vi "HFRR ADV v08.vi"() -> ()   [LabVIEW 2025] (continued)
          frame True {
            (unwired) 0  # existing file
            w3721 = "Choose a datalog file to open"  # prompt
            n2718 = local write "OPEN 3"(FALSE ("OPEN 1")) -> ()
            n2719 = String To Path(string="C:\\LAB-IQ\\Data\\") -> (path=w3706:path)
            n2720 = File Dialog(6:"*.dgf" ("pattern"), 7:w3721, 11:w3706) -> (0:w3704:errorcluster, 3:w3712:path)  [unwired: 4 in, 2 out]
            n2721 = Unbundle(w3704) -> ()  [unwired: 3 out]
            n2722 = Strip Path(path=w3712) -> (name=w3710:string)  [unwired: 1 out]
            n2723 = Path To String(path=w3712) -> (string=w3707:string)
            "string1 3" <- w3707
            n2724 = Match Pattern(string=w3710, regular expression=".dgf") -> (before substring=→"String Control 5":string)  [unwired: 1 in, 3 out]
            n2725 = Match Pattern(string=w3707, regular expression=".dgf" ("substring (\"\")")) -> (before substring=w3717:string)  [unwired: 1 in, 3 out]
            n2726 = Concatenate Strings(w3717, ".duf" ("Substring")) -> (w3714:string)
            n2727 = String To Path(string=w3714) -> (path=w3718:path)
            n2728 = call <vilib>:"Read Characters From File.vi"("file path (dialog if empty)"=w3718, "start of read offset (chars.:0)"=60 ("start of read offset (chars.: 0)")) -> ("character string"=→"String Control 6":string)  [unwired: 4 in, 3 out]
          }
        }
        n2729 = case shown="True" "OPEN 4" {
          frame False {
          }
          frame True {
            (unwired) 0  # existing file
            w3739 = "Choose a datalog file to open"  # prompt
            n2730 = local write "OPEN 4"(FALSE ("OPEN 1")) -> ()
            n2731 = String To Path(string="C:\\LAB-IQ\\Data\\") -> (path=w3724:path)
            n2732 = File Dialog(6:"*.dgf" ("pattern"), 7:w3739, 11:w3724) -> (0:w3722:errorcluster, 3:w3730:path)  [unwired: 4 in, 2 out]
            n2733 = Unbundle(w3722) -> ()  [unwired: 3 out]
            n2734 = Strip Path(path=w3730) -> (name=w3728:string)  [unwired: 1 out]
            n2735 = Path To String(path=w3730) -> (string=w3725:string)
            "string1 4" <- w3725
            n2736 = Match Pattern(string=w3728, regular expression=".dgf") -> (before substring=→"String Control 7":string)  [unwired: 1 in, 3 out]
            n2737 = Match Pattern(string=w3725, regular expression=".dgf" ("substring (\"\")")) -> (before substring=w3735:string)  [unwired: 1 in, 3 out]
            n2738 = Concatenate Strings(w3735, ".duf" ("Substring")) -> (w3732:string)
            n2739 = String To Path(string=w3732) -> (path=w3736:path)
            n2740 = call <vilib>:"Read Characters From File.vi"("file path (dialog if empty)"=w3736, "start of read offset (chars.:0)"=60 ("start of read offset (chars.: 0)")) -> ("character string"=→"String Control 8":string)  [unwired: 4 in, 3 out]
          }
        }
      }
      frame "About" {
        # "Elapsed time\ncof\nstroke\nmean pos\nTemp\nHumidity"
        n2741 = disable-structure shown="Disabled" {
          frame Disabled {
            n2742 = case shown="True" "Export" {
              frame False {
              }
              frame True {
                w3761 = "                                      " ("string")
                w3763 = "\r"
                (unwired) i16 6 ("width (-)")
                w3840 = "\r"
                w3772 = "\r"
                n2743 = local write "Export"(FALSE ("Export")) -> ()
                n2744 = local read "String 29"() -> (w3809:string)
                n2745 = local read "String 34"() -> (w3797:string)
                n2746 = local read "String 35"() -> (w3792:string)
                n2747 = local read "String 37"() -> (w3788:string)
                n2748 = local read "String 36"() -> (w3785:string)
                n2749 = local read "String 38"() -> (w3782:string)
                n2750 = local read "String 39"() -> (w3779:string)
                n2751 = Match Pattern(string=w3809, regular expression=".dwm") -> (before substring=w3805:string)  [unwired: 1 in, 3 out]
                "before substring" <- w3805
                n2752 = local read "S 38"() -> (w3800:string)
                n2753 = local read "S 39"() -> (w3793:string)
                n2754 = local read "Temperature before test 2"() -> (w3829:dbl)
                n2755 = local read "Temperature after test 2"() -> (w3834:dbl)
                n2756 = local read "Humidity before test 2"() -> (w3815:dbl)
                n2757 = local read "Humidity after test 2"() -> (w3830:dbl)
                n2758 = local read "MWSD 2"() -> (w3826:dbl)
                n2759 = local read "WS1.4 2"() -> (w3842:dbl)
                n2760 = local read "HCF 2"() -> (w3838:dbl)
                n2761 = local read "AVP 2"() -> (w3827:dbl)
                n2762 = Concatenate Strings("1," ("string"), w3800) -> (w3799:string)
                n2763 = Concatenate Strings("2," ("string"), w3797) -> (w3796:string)
                n2764 = Concatenate Strings("3," ("string"), w3793) -> (w3795:string)
                n2765 = Concatenate Strings("4," ("string"), w3792) -> (w3791:string)
                n2766 = Concatenate Strings("5," ("string"), w3788) -> (w3789:string)
                n2767 = Concatenate Strings("6," ("string"), w3785) -> (w3786:string)
                n2768 = Concatenate Strings("7," ("string"), w3782) -> (w3783:string)
                n2769 = Concatenate Strings("8," ("string"), w3779) -> (w3780:string)
                n2770 = local read "Sample ID"() -> (w3847:string)
                n2771 = case shown="\"xlx\"" "Select File Type" {
                  tunnel: w3805 -> [w3850 w3852 w3854]
                  tunnel: [w3848 w3853 w3855] -> w3804
                  frame "xlx" {
                    n2772 = Concatenate Strings(w3850, ".xls" ("string")) -> (w3848:string)
                  }
                  frame "csv" {
                    n2773 = Concatenate Strings(w3852, ".csv" ("string")) -> (w3853:string)
                  }
                  frame "txt" {
                    n2774 = Concatenate Strings(w3854, ".txt" ("string")) -> (w3855:string)
                  }
                }
                n2775 = local read "Test Date"() -> (w3846:string)
                n2776 = local read "String 45"() -> (w3760:string)
                n2777 = local read "String 31"() -> (w3845:string)
                n2778 = local read "String 32"() -> (w3844:string)
                n2779 = local read "TITTLE"() -> (w3768:string)
                n2780 = Number To Fractional String(number=w3815, width (-)=i16 6, precision (6)=i16 2) -> (F-format string=w3814:string)  [unwired: 1 in]
                n2781 = Number To Fractional String(number=w3829, width (-)=i16 6, precision (6)=i16 2) -> (F-format string=w3835:string)  [unwired: 1 in]
                n2782 = Number To Fractional String(number=w3830, width (-)=i16 6, precision (6)=i16 2) -> (F-format string=w3828:string)  [unwired: 1 in]
                n2783 = Number To Fractional String(number=w3834, width (-)=i16 6, precision (6)=i16 2) -> (F-format string=w3833:string)  [unwired: 1 in]
                n2784 = Number To Fractional String(number=w3826, width (-)=i16 6, precision (6)=i16 2) -> (F-format string=w3824:string)  [unwired: 1 in]
                n2785 = Number To Fractional String(number=w3827, width (-)=i16 6, precision (6)=i16 2) -> (F-format string=w3825:string)  [unwired: 1 in]
                n2786 = Number To Fractional String(number=w3838, width (-)=i16 6, precision (6)=i16 2) -> (F-format string=w3839:string)  [unwired: 1 in]
                n2787 = Number To Fractional String(number=w3842, precision (6)=i16 2) -> (F-format string=w3843:string)  [unwired: 2 in]
                n2788 = local read "s.NO"() -> (w3762:string)
                n2789 = Concatenate Strings("=" ("string"), w3768) -> (w3767:string)
                n2790 = Concatenate Strings("S.No," ("string"), "                                       Parameters" ("string")) -> (w3773:string)
                n2791 = Concatenate Strings(w3840, w3799, w3814, w3840, w3796, w3835, w3840, w3795, w3828, w3840, w3791, w3833, w3840, w3789, w3824, w3840, w3786, w3825, w3840, w3783, w3839, w3840, w3780, w3843) -> (w3802:string)
                n2792 = Concatenate Strings(w3772, "," ("string"), w3760, w3762, w3761, w3844, w3847, w3761, w3845, w3846, w3772) -> (w3770:string)
                n2793 = local read "Tested by"() -> (w3776:string)
                n2794 = local read "String 33"() -> (w3777:string)
                n2795 = Concatenate Strings("," ("string"), "                                                                             " ("string")) -> (w3765:string)
                n2796 = Concatenate Strings(w3767, w3763, w3770, w3763, w3773, w3802, w3763, w3765, w3777, w3776) -> (→"export":string)
                n2797 = String To Path(string=w3804) -> (path=w3811:path)
                n2798 = local read "export"() -> (w3806:string)
                n2799 = call <vilib>:"Write Characters To File.vi"("append to file? (new file:F)"=FALSE, "character string"=w3806, "file path (dialog if empty)"=w3811) -> ()  [unwired: 2 in, 1 out]
              }
            }
          }
          frame Enabled {
          }
        }
        n2800 = case shown="True" "OK Button 17" {
          frame False {
          }
          frame True {
            (unwired) 0  # existing file
            w4064 = "Choose a datalog file to open"  # prompt
            n2801 = local write "OK Button 17"(FALSE ("OK Button 17")) -> ()
            n2802 = local read "String"() -> (w4059:string)
            n2803 = String To Path(string=w4059) -> (path=w4060:path)
            n2804 = File Dialog(6:"*.duf" ("pattern"), 7:w4064, 11:w4060) -> (0:w4051:errorcluster, 3:w4070:path)  [unwired: 4 in, 2 out]
            n2805 = Unbundle(w4051) -> ()  [unwired: 3 out]
            n2806 = Open/Create/Replace File "Open File"(file path (use dialog)=w4070) -> (refnum out=w4062:refnum<file>)  [unwired: 5 in, 2 out]
            n2807 = Strip Path(path=w4070) -> (name=w4068:string)  [unwired: 1 out]
            n2808 = Path To String(path=w4070) -> (string=w4053:string)
            n2809 = while {
              tunnel: w4062 -> [w4074]
              i -> [w4071]
              stop <- w4072 continue-if-true
              (unwired) TRUE ("line mode (F)")
              n2810 = Read from Text File "Read File"(file (use dialog)=w4074) -> (text=w4073:string)  [unwired: 3 in, 3 out]
              n2811 = local write "Numeric 16"(w4071) -> ()
              n2812 = String Length(string=w4073) -> (length=w4076:i32)
              n2813 = Greater?(x=w4076, y=1) -> (0:w4072:bool)
            }
            n2814 = local write "String 29"(w4053) -> ()
            n2815 = Search and Replace String(input string=w4053, search string=".duf", replace string=".dgf" ("replace string (\"\")")) -> (result string=→"String Indicator 4":string)  [unwired: 5 in, 3 out]
            n2816 = Match Pattern(string=w4068, regular expression=".dwm") -> (before substring=w4052:string)  [unwired: 1 in, 3 out]
            "String Indicator" <- w4052
            n2817 = Match Pattern(string=w4053, regular expression=".dwm" ("substring (\"\")")) -> (before substring=w4054:string)  [unwired: 1 in, 3 out]
            "String Indicator 3" <- w4054
            n2818 = local write "TITTLE 2"(w4052) -> ()
            n2819 = String To Path(string=w4054) -> (path=w4061:path)
            "path" <- w4061
            n2820 = call <vilib>:"Read Characters From File.vi"("file path (dialog if empty)"=w4061, "start of read offset (chars.:0)"=60 ("start of read offset (chars.: 0)")) -> ("character string"=→"String Indicator 2":string)  [unwired: 4 in, 3 out]
          }
        }
        n2821 = call <vilib>:"Query Available Printers.vi"() -> ("system configured printers"=w3753:string[])  [unwired: 9 in, 2 out]
        "System Configured Printers 2" <- w3753
        n2822 = local read "OK Button 16"() -> (w3750:bool)
        n2823 = case shown="True" "OK Button 16" {
          frame False {
          }
          frame True {
            n2824 = stacked-sequence {
              frame #0 {
                n2825 = local read "Numeric 16"() -> (w4078:i32)
                n2826 = local write "Numeric 10"(w4078) -> ()
              }
              frame #1 {
                n2827 = local read "S.NO"() -> (→"s.NO":string)
                n2828 = local read "String 29"() -> (w4082:string)
                n2829 = String To Path(string=w4082) -> (path=w4081:path)
                n2830 = Open/Create/Replace File "Open File"(file path (use dialog)=w4081) -> (refnum out=w4083:refnum<file>)  [unwired: 5 in, 2 out]
                n2831 = for {
                  N: 16 -> [_]
                  tunnel: w4083 -> [w4090]
                  i -> [w4086]
                  (unwired) TRUE ("line mode (F)")
                  n2832 = Read from Text File "Read File"(file (use dialog)=w4090) -> (text=w4084:string)  [unwired: 3 in, 3 out]
                  n2833 = Match Pattern(string=w4084, regular expression="(") -> (after substring=w4089:string)  [unwired: 1 in, 3 out]
                  n2834 = Match Pattern(string=w4089, regular expression=")") -> (before substring=w4085:string)  [unwired: 1 in, 3 out]
                  n2835 = case shown="1" w4086 {
                    tunnel: w4085 -> [w4091 w4092 _ _ w4093 w4094 w4095 w4097 w4099 w4101 w4103 w4105 w4107 w4109 _]
                    tunnel: w4084 -> [_ _ _ _ _ _ _ _ _ _ _ _ _ _ _]
                    frame 0 {
                      "TITTLE" <- w4091
                    }
                    frame 1 {
                      "Sample ID" <- w4092
                    }
                    frame 2 {
                    }
                    frame 3 {
                    }
                    frame 4 {
                      "Test Date" <- w4093
                    }
                    frame 5 {
                      "Tested by" <- w4094
                    }
                    frame 6 {
                      n2836 = Fract/Exp String To Number(string=w4095) -> (number=→"Humidity before test 2":dbl)  [unwired: 3 in, 1 out]
                    }
                    frame 7 {
                      n2837 = Fract/Exp String To Number(string=w4097) -> (number=→"Temperature before test 2":dbl)  [unwired: 3 in, 1 out]
                    }
                    frame 8 {
                      n2838 = Fract/Exp String To Number(string=w4099) -> (number=→"Humidity after test 2":dbl)  [unwired: 3 in, 1 out]
                    }
                    frame 9 {
                      n2839 = Fract/Exp String To Number(string=w4101) -> (number=→"Temperature after test 2":dbl)  [unwired: 3 in, 1 out]
                    }
                    frame 10 {
                      n2840 = Fract/Exp String To Number(string=w4103) -> (number=→"MWSD 2":dbl)  [unwired: 3 in, 1 out]
                    }
                    frame 11 {
                      n2841 = Fract/Exp String To Number(string=w4105) -> (number=→"AVP 2":dbl)  [unwired: 3 in, 1 out]
                    }
                    frame 12 {
                      n2842 = Fract/Exp String To Number(string=w4107) -> (number=→"HCF 2":dbl)  [unwired: 3 in, 1 out]
                    }
                    frame 13 {
                      n2843 = Fract/Exp String To Number(string=w4109) -> (number=→"WS1.4 2":dbl)  [unwired: 3 in, 1 out]
                    }
                    frame 14, Default {
                    }
                  }
                }
              }
              frame #2 {
              }
            }
            n2844 = local write "OK Button 16"(FALSE ("OK Button 13")) -> ()
          }
        }
        n2845 = Index Array(array=w3753, index="Select Printer 3") -> (element=w3755:string)
        "Selected Printer" <- w3755
        n2846 = case shown="True" w3750 {
          frame False {
          }
          frame True {
            n2847 = flat-sequence {
              frame #0 {
              }
              frame #1 {
                n2848 = Wait (ms)(milliseconds to wait=u32 100) -> ()  [unwired: 1 out]
              }
              frame #2 {
                n2849 = local write "OK Button 16"(FALSE ("Print 3")) -> ()
              }
            }
          }
        }
        n2850 = case shown="True" "Print" {
          tunnel: w3755 -> [_ w4047]
          frame False {
          }
          frame True {
            (unwired) i16 6 ("width (-)")
            (unwired) "TESTED BY : "
            (unwired) "TESTED DATE :"
            (unwired) "SAMPLE ID : "
            (unwired) "SAMPLE DESIGN : "
            w4005 = "\r"
            w4022 = "\r"
            # "add image"
            n2851 = local read "Sample ID"() -> (w3995:string)
            n2852 = local read "Tested by"() -> (w3998:string)
            n2853 = local read "String 34"() -> (w3985:string)
            n2854 = local read "String 45"() -> (w3965:string)
            n2855 = local read "String 35"() -> (w3980:string)
            n2856 = local read "String 37"() -> (w3978:string)
            n2857 = local read "String 32"() -> (w4000:string)
            n2858 = local read "String 36"() -> (w3975:string)
            n2859 = local read "String 31"() -> (w3999:string)
            n2860 = local read "Test Date"() -> (w3996:string)
            n2861 = local read "String 33"() -> (w4001:string)
            n2862 = local read "String 38"() -> (w3971:string)
            n2863 = local read "String 39"() -> (w3968:string)
            n2864 = local write "Print"(FALSE ("Print FF")) -> ()
            n2865 = local read "S 39"() -> (w3983:string)
            n2866 = local read "S 38"() -> (w3990:string)
            n2867 = local read "Temperature before test 2"() -> (w4021:dbl)
            n2868 = local read "Temperature after test 2"() -> (w4011:dbl)
            n2869 = local read "Humidity before test 2"() -> (w4036:dbl)
            n2870 = local read "Humidity after test 2"() -> (w4020:dbl)
            n2871 = local read "MWSD 2"() -> (w4025:dbl)
            n2872 = local read "WS1.4 2"() -> (w4003:dbl)
            n2873 = Concatenate Strings("2)" ("string"), w3985) -> (w3986:string)
            n2874 = Concatenate Strings("3)" ("string"), w3983) -> (w3984:string)
            n2875 = Concatenate Strings("1)" ("string"), w3990) -> (w3989:string)
            n2876 = Concatenate Strings("4)" ("string"), w3980) -> (w3981:string)
            n2877 = Concatenate Strings("5)" ("string"), w3978) -> (w3977:string)
            n2878 = Concatenate Strings("6)" ("string"), w3975) -> (w3974:string)
            n2879 = Concatenate Strings("7)" ("string"), w3971) -> (w3972:string)
            n2880 = Concatenate Strings("8)" ("string"), w3968) -> (w3969:string)
            n2881 = local read "HCF 2"() -> (w4007:dbl)
            n2882 = local read "AVP 2"() -> (w4024:dbl)
            n2883 = local read "s.NO"() -> (w3966:string)
            n2884 = call <vilib>:"New Report.vi"("report type"=enum16{"Standard Report", "HTML"}."Standard Report") -> ("report out"=w4045:refnum<class "NI_report.lvclass">, "error out"=w4044:errorcluster)  [unwired: 13 in]
            n2885 = local read "TITTLE"() -> (w3997:string)
            n2886 = Concatenate Strings(w4022, w3965, w3966, w4022, w4000, w3995, w4022, w3999, w3996, w4022, w4001, w3998, w4022) -> (w4015:string)
            "test by" <- w4015
            n2887 = Number To Fractional String(number=w4021, width (-)=i16 6, precision (6)=i16 2) -> (F-format string=w4010:string)  [unwired: 1 in]
            n2888 = Number To Fractional String(number=w4020, width (-)=i16 6, precision (6)=i16 2) -> (F-format string=w4023:string)  [unwired: 1 in]
            n2889 = Number To Fractional String(number=w4036, width (-)=i16 6, precision (6)=i16 2) -> (F-format string=w4041:string)  [unwired: 1 in]
            n2890 = Number To Fractional String(number=w4025, width (-)=i16 6, precision (6)=i16 2) -> (F-format string=w4027:string)  [unwired: 1 in]
            n2891 = Number To Fractional String(number=w4011, width (-)=i16 6, precision (6)=i16 2) -> (F-format string=w4012:string)  [unwired: 1 in]
            n2892 = Number To Fractional String(number=w4024, width (-)=i16 6, precision (6)=i16 2) -> (F-format string=w4026:string)  [unwired: 1 in]
            n2893 = Number To Fractional String(number=w4007, width (-)=i16 6, precision (6)=i16 2) -> (F-format string=w4006:string)  [unwired: 1 in]
            n2894 = Number To Fractional String(number=w4003, precision (6)=i16 2) -> (F-format string=w4002:string)  [unwired: 2 in]
            n2895 = call-dynamic "Set Report Header Text.vi"("report in"=w4045, "center header text"=w3997, "error in (no error)"=w4044) -> ("report out"=w4016:refnum<class "NI_report.lvclass">, "error out"=w4017:errorcluster)  [unwired: 11 in]
            n2896 = Concatenate Strings(w4005, w3989, w4041, w4005, w3986, w4010, w4005, w3984, w4023, w4005, w3981, w4012, w4005, w3977, w4027, w4005, w3974, w4026, w4005, w3972, w4006, w4005, w3969, w4002) -> (w3993:string)
            "export 2" <- w3993
            n2897 = call-poly <vilib>:"Append Report Text.vi"("report in"=w4016, "text"=w4015, "error in (no error)"=w4017) -> ("report out"=w4019:refnum<class "NI_report.lvclass">, "error out"=w4018:errorcluster)  [unwired: 9 in, 2 out]
            n2898 = local read "test by"() -> (w3992:string)
            n2899 = local read "TITTLE"() -> (w3994:string)
            n2900 = call-poly <vilib>:"Append Report Text.vi"("report in"=w4019, "error in (no error)"=w4018) -> ("report out"=w4040:refnum<class "NI_report.lvclass">, "error out"=w4038:errorcluster)  [unwired: 10 in, 2 out]
            n2901 = Concatenate Strings(w3994, w3993, w3992) -> (→"output":string)
            n2902 = call-poly <vilib>:"Append Report Text.vi"("report in"=w4040, "text"=w3993, "error in (no error)"=w4038) -> ("report out"=w4039:refnum<class "NI_report.lvclass">, "error out"=w4037:errorcluster)  [unwired: 9 in, 2 out]
            n2903 = call-dynamic "Print Report.vi"("report in"=w4039, "printer name (default)"=w4047, "error in (no error)"=w4037) -> ("report out"=w4049:refnum<class "NI_report.lvclass">, "error out"=w4050:errorcluster)  [unwired: 11 in]
            n2904 = call-dynamic "Dispose Report.vi"("report in"=w4049, "error in (no error)"=w4050) -> ()  [unwired: 13 in, 1 out]
          }
        }
        n2905 = case shown="True" "Print 2" {
          frame False {
          }
          frame True {
            n2906 = flat-sequence {
              frame #0 {
                n2907 = local read "s.NO"() -> (→"s.NO 2":string)
                n2908 = Wait (ms)(milliseconds to wait=u32 20) -> ()  [unwired: 1 out]
                n2909 = local read "Sample ID  3"() -> (→"Sample ID  6":string)
                n2910 = local read "Sample ID  4"() -> (→"Sample ID  7":string)
                n2911 = local read "Sample ID"() -> (→"Sample ID  2":string)
                n2912 = local read "Tested by"() -> (→"Tested by 2":string)
                n2913 = local read "Test Date"() -> (→"Test Date 2":string)
                n2914 = local read "Humidity after test 3"() -> (→"Humidity after test 4":dbl)
                n2915 = local read "Ref A Test Date :"() -> (→"TITTLE 4":string)
                n2916 = local read "Temperature before test 3"() -> (w3872:dbl)
                n2917 = local read "Temperature before test 3"() -> (→"Temperature after test 5":dbl)
                n2918 = local read "Temperature after test 3"() -> (→"Temperature after test 4":dbl)
                n2919 = local read "Humidity before test 3"() -> (→"Humidity before test 4":dbl)
                n2920 = local write "Temperature before test 3"(w3872) -> ()
                n2921 = local read "image data"() -> (w3863:T12)
                n2922 = String To Path(string="C:\\LAB-IQ\\im\\Temp_resized.jpg") -> (path=w3864:path)
                "path 2" <- w3864
                n2923 = call <vilib>:"Write JPEG File.vi"("image data"=w3863, "path to JPEG file"=w3864) -> ()  [unwired: 8 in, 2 out]
                "Ref A Test Date :" <- "Ref A Test Date :"
                "Ref B Test Date :" <- "Ref B Test Date :"
                "Ref B Scar Value :" <- "Ref B Scar Value :"
                "Ref A Scar Value :" <- "Ref A Scar Value :"
              }
              frame #1 {
                (unwired) HTML_Report_Image_Alignment."MIDDLE" ("alignment (default)")
                w3900 = u16 0 items=["portrait", "landscape"] ("orientation (portrait)")
                (unwired) HTML_Report_Image_Alignment."ABSMIDDLE" ("alignment (default)")
                (unwired) "TESTED BY : "
                (unwired) "TESTED DATE :"
                (unwired) "SAMPLE ID : "
                (unwired) "SAMPLE DESIGN : "
                w3933 = "\r"
                # "add image"
                n2924 = Wait (ms)(milliseconds to wait=u32 20) -> ()  [unwired: 1 out]
                n2925 = local read "Sample ID  2"() -> (w3926:string)
                n2926 = local read "Wear Scar X"() -> (w3898:dbl)
                "Length ( microns ) 2" <- w3898
                n2927 = local read "Wear Scar Y"() -> (w3897:dbl)
                "Wear Scar Y ( microns ) :" <- w3897
                n2928 = local read "Test Date 2"() -> (w3927:string)
                n2929 = local read "Tested by 2"() -> (w3928:string)
                n2930 = local read "String 46"() -> (w3924:string)
                n2931 = local read "String 48"() -> (w3930:string)
                n2932 = local read "String 47"() -> (w3929:string)
                n2933 = local read "String 49"() -> (w3931:string)
                n2934 = local read "String 10"() -> (w3884:string)
                n2935 = local read "s.NO 2"() -> (w3925:string)
                n2936 = Add(x=w3898, y=w3897) -> (x+y=w3896:dbl)
                n2937 = call <vilib>:"New Report.vi"("report type"=enum16{"Standard Report", "HTML"}."HTML") -> ("report out"=w3904:refnum<class "NI_report.lvclass">, "error out"=w3902:errorcluster)  [unwired: 13 in]
                n2938 = Concatenate Strings(w3933, w3924, w3925, w3933, w3930, w3926, w3933, w3929, w3927, w3933, w3931, w3928, w3933) -> (→"test by 2":string)
                n2939 = Concatenate Strings("C:\\LAB-IQ\\Data\\" ("string"), w3884, ".jpg" ("string")) -> ()  [unwired: 1 out]
                n2940 = Divide(x=w3896, y=2.0) -> (x/y=→"Mean Wear ( microns) :":dbl)
                n2941 = call-dynamic "Set Report Orientation.vi"("report in"=w3904, "orientation (portrait)"=w3900, "error in (no error)"=w3902) -> ("report out"=w3903:refnum<class "NI_report.lvclass">, "error out"=w3901:errorcluster)  [unwired: 11 in]
                n2942 = for {
                  N: 5 -> [_]
                  tunnel: w3903 -> [w3954]
                  tunnel: [w3953] -> w3882
                  tunnel: w3901 -> [w3952]
                  tunnel: [w3951] -> w3881
                  n2943 = call-dynamic "Set Report Tab Width.vi"("report in"=w3954, "error in (no error)"=w3952) -> ("report out"=w3953:refnum<class "NI_report.lvclass">, "error out"=w3951:errorcluster)  [unwired: 12 in]
                }
                n2944 = local read "TITTLE"() -> (w3899:string)
                n2945 = call-dynamic "Set Report Header Text.vi"("report in"=w3882, "center header text"=w3899, "error in (no error)"=w3881) -> ("report out"=w3920:refnum<class "NI_report.lvclass">, "error out"=w3919:errorcluster)  [unwired: 11 in]
                n2946 = for {
                  N: 1 -> [_]
                  tunnel: [w3958] -> w3906
                  tunnel: [w3957] -> w3905
                  tunnel: w3920 -> [w3956]
                  tunnel: w3919 -> [w3955]
                  n2947 = call-dynamic "New Report Line.vi"("report in"=w3956, "error in (no error)"=w3955) -> ("report out"=w3958:refnum<class "NI_report.lvclass">, "error out"=w3957:errorcluster)  [unwired: 12 in]
                }
                n2948 = for {
                  N: 2 -> [_]
                  tunnel: [w3950] -> w3912
                  tunnel: [w3949] -> w3911
                  tunnel: w3906 -> [w3948]
                  tunnel: w3905 -> [w3947]
                  n2949 = call-dynamic "New Report Line.vi"("report in"=w3948, "error in (no error)"=w3947) -> ("report out"=w3950:refnum<class "NI_report.lvclass">, "error out"=w3949:errorcluster)  [unwired: 12 in]
                }
                n2950 = for {
                  N: 25 -> [_]
                  tunnel: w3912 -> [w3946]
                  tunnel: w3911 -> [w3944]
                  tunnel: [w3945] -> w3915
                  tunnel: [w3943] -> w3914
                  n2951 = call-dynamic "Set Report Tab Width.vi"("report in"=w3946, "error in (no error)"=w3944) -> ("report out"=w3945:refnum<class "NI_report.lvclass">, "error out"=w3943:errorcluster)  [unwired: 12 in]
                }
                n2952 = control-ref of="Tab Control 9"() -> (w3910:refnum<vi>)
                n2953 = call-dynamic "Append Control Image to Report.vi"("report in"=w3915, "alignment (default)"=HTML_Report_Image_Alignment."ABSMIDDLE", "ctrl reference"=w3910, "error in (no error)"=w3914) -> ("report out"=w3909:refnum<class "NI_report.lvclass">, "error out"=w3908:errorcluster)  [unwired: 8 in, 2 out]
                n2954 = for {
                  N: 3 -> [_]
                  tunnel: [w3942] -> w3893
                  tunnel: [w3941] -> w3892
                  tunnel: w3909 -> [w3940]
                  tunnel: w3908 -> [w3939]
                  n2955 = call-dynamic "New Report Line.vi"("report in"=w3940, "error in (no error)"=w3939) -> ("report out"=w3942:refnum<class "NI_report.lvclass">, "error out"=w3941:errorcluster)  [unwired: 12 in]
                }
                n2956 = for {
                  N: 100 -> [_]
                  tunnel: w3893 -> [w3938]
                  tunnel: w3892 -> [w3936]
                  tunnel: [w3937] -> w3889
                  tunnel: [w3935] -> w3887
                  n2957 = call-dynamic "Set Report Tab Width.vi"("report in"=w3938, "error in (no error)"=w3936) -> ("report out"=w3937:refnum<class "NI_report.lvclass">, "error out"=w3935:errorcluster)  [unwired: 12 in]
                }
                n2958 = String To Path(string="C:\\LAB-IQ\\im\\Temp_resized.jpg") -> (path=w3879:path)
                n2959 = call-poly <vilib>:"Append Image to Report.vi"("report in"=w3889, "path or URL of image"=w3879, "error in (no error)"=w3887) -> ("report out"=w3888:refnum<class "NI_report.lvclass">, "error out"=w3886:errorcluster)  [unwired: 9 in, 2 out]
                n2960 = call-poly <vilib>:"Open HTML Report in Browser.vi"("report in"=w3888, "error in (no error)"=w3886) -> ("report out"=w3923:refnum<class "NI_report.lvclass">, "error out"=w3922:errorcluster)  [unwired: 11 in, 1 out]
                n2961 = call-dynamic "Dispose Report.vi"("report in"=w3923, "error in (no error)"=w3922) -> ()  [unwired: 13 in, 1 out]
              }
              frame #2 {
              }
              frame #3 {
                n2962 = disable-structure shown="Disabled" {
                  frame Disabled {
                    n2963 = local read "String 10"() -> (w3963:string)
                    n2964 = Concatenate Strings("C:\\LAB-IQ-NXT\\Data\\" ("string"), w3963, ".jpg" ("string")) -> (w3961:string)
                    n2965 = String To Path(string=w3961) -> (path=w3960:path)
                    n2966 = Delete(path (use dialog)=w3960) -> ()  [unwired: 4 in, 3 out]
                  }
                  frame Enabled {
                  }
                }
                n2967 = local write "Print 2"(FALSE ("Print")) -> ()
              }
            }
          }
        }
      }
    }
    n2968 = property on="SetTemp" class="DigNum (strict)"("Disabled"=w1894) -> ()  [unwired: 2 in, 2 out]
    n2969 = Multiply(x=w1883, y=w1885) -> (x*y=w1884:dbl)
    n2970 = local read "MWSD"() -> (w1882:dbl)
    n2971 = Add(x=w1884, y=w1882) -> (x+y=→"WS1.4":dbl)
    n2972 = Wait (ms)(milliseconds to wait=u32 50) -> ()  [unwired: 1 out]
    n2973 = Wait (ms)(milliseconds to wait=u32 50) -> ()  [unwired: 1 out]
    n2974 = local read "Quit"() -> (w1881:bool)
  }
  n2975 = VISA Close(VISA resource name=w46, error in (no error)=w45) -> (error out=w43:errorcluster)
  n2976 = VISA Close(VISA resource name=w27, error in (no error)=w26) -> ()  [unwired: 1 out]
  n2977 = call <vilib>:"Clear Errors.vi"("error in (no error)"=w43) -> ()  [unwired: 5 in, 2 out]
  n2978 = Or(x=w33, y=w32) -> (x .or. y?=w34:bool)
  n2979 = while {
    tunnel: [w4111] -> w39
    shift-right: [w4149] -> _
    shift-left: "" -> [w4137]
    tunnel: [w4125] -> _
    i -> [w4125]
    stop <- w4111 stop-if-true
    w4151 = ";" ("string")
    n2980 = local read "start en"() -> (w4170:bool)
    n2981 = And(x="st enable", y=w4170) -> (x .and. y?=w4171:bool)
    n2982 = local read "ACQUIRE 3"() -> (w4114:bool)
    n2983 = local read "Elapsed time"() -> (w4133:dbl)
    n2984 = case shown="True" w4171 {
      tunnel: "st enable" -> [w4235 w4236]
      tunnel: [w4235 w4236] -> w4115
      frame False {
      }
      frame True {
        n2985 = local write "start en"(FALSE ("start en")) -> ()
      }
    }
    n2986 = Wait (ms)(milliseconds to wait=u32 80) -> ()  [unwired: 1 out]
    n2987 = local read "Stroke"() -> (w4124:dbl)
    n2988 = Greater?(x=w4133, y=0.1) -> (0:w4131:bool)
    n2989 = Or(x=w4115, y=w4114) -> (x .or. y?=w4116:bool)
    n2990 = case shown="True" "ACQUIRE 2" {
      frame False {
      }
      frame True {
        n2991 = call "Elapsed Time13"() -> ("Time has Elapsed"=w4178:bool)  [unwired: 12 in, 7 out]
        n2992 = case shown="True" w4178 {
          frame False {
          }
          frame True {
            n2993 = local write "ACQUIRE 2"(FALSE ("ACQUIRE 2")) -> ()
            n2994 = local write "ACQUIRE 3"(FALSE ("ACQUIRE 2")) -> ()
          }
        }
        n2995 = local write "ACQUIRE 3"(TRUE ("ACQUIRE 2")) -> ()
      }
    }
    n2996 = case shown="True" w4116 {
      tunnel: w4124 -> [_ w4258]
      tunnel: [w4238 _] -> w4168
      tunnel: w4131 -> [_ _]
      tunnel: w4114 -> [_ w4245]
      frame False {
        w4238 = TRUE ("PID Rst")
        n2997 = local read "stop cmd"() -> (w4239:bool)
        n2998 = case shown="True" w4239 {
          frame False {
          }
          frame True {
            n2999 = local write "stop cmd"(FALSE ("stop cmd")) -> ()
          }
        }
        n3000 = local write "PID Rst"(TRUE ("PID Rst")) -> ()
        "start en" <- w4238
      }
      frame True {
        w4265 = cluster{"output high":dbl, "output low":dbl} {"output high"=600.0, "output low"=-600.0} ("output range")
        n3001 = local read "STROKE GAIN :"() -> (w4250:dbl)
        n3002 = call "Elapsed Time6"("Reset"="PID Rst", "Auto Reset"=FALSE) -> ("Time has Elapsed"=w4259:bool)  [unwired: 10 in, 7 out]
        n3003 = Multiply(x="Set Strk", y=w4250) -> (x*y=w4243:dbl)
        n3004 = case shown="False" w4259 {
          tunnel: [w4270 w4271] -> w4262
          tunnel: "Set Strk" -> [w4270 _]
          tunnel: w4258 -> [_ w4271]
          frame False {
          }
          frame True {
          }
        }
        n3005 = Multiply(x=w4243, y=1.0) -> (x*y=w4242:dbl)
        n3006 = Select(t=T9 {"Proportional Gain (Kc)"=0.0, "Integral Time (Ti, min)"=0.02, "Derivative Time (Td, min)"=0.0} ("Stroke PID Gains"), s=w4245, f="Stroke PID Gains") -> (s? t:f=w4246:T9)
        n3007 = Not(x=w4259) -> (.not. x?=w4257:bool)
        n3008 = call-poly <vilib>:"PID.vi"("reinitialize? (F)"=w4257, "output range"=w4265, "PID gains"=w4246, "process variable"=w4262, "setpoint"="Set Strk") -> ("output"=w4256:dbl)  [unwired: 5 in, 1 out]
        "Stroke PID OUT" <- w4256
        n3009 = Select(t=w4256, s=w4259, f=0.0) -> (s? t:f=w4260:dbl)
        n3010 = flat-sequence {
          tunnel: w4260 -> [_]
          frame #0 {
            n3011 = local write "PID Rst"(FALSE ("PID Rst")) -> ()
          }
        }
        n3012 = Add(x=w4242, y=w4260) -> (x+y=w4255:dbl)
        n3013 = Unbundle(w4265) -> ("output high"=w4264:dbl, "output low"=w4263:dbl)
        n3014 = To Word Integer(number=w4255) -> (16bit integer=w4252:i16)
        n3015 = property on="Stroke PID OUT" class="Slide (strict)"("Scale.Range:Minimum"=w4263, "Scale.Range:Maximum"=w4264) -> ()  [unwired: 2 in, 2 out]
        n3016 = In Range and Coerce(upper limit=4095.0 ("f"), x=w4252, lower limit=100.0 ("f")) -> (coerced(x)=w4249:dbl)  [unwired: 1 out]
        "PID Out" <- w4249
        n3017 = Number To Decimal String(number=w4249) -> (decimal integer string=→"st gain":string)  [unwired: 1 in]
        "stop cmd" <- TRUE ("Auto Reset")
      }
    }
    n3018 = flat-sequence {
      frame #0 {
        n3019 = local read "CH-POWER +"() -> (w4182:u16)
        n3020 = local read "CH-POWER -"() -> (w4183:u16)
        n3021 = case shown="1" w4183 {
          tunnel: "PWR" -> [w4184 w4185 w4186 w4187 w4188 w4189 w4190 w4191]
          frame 0, Default {
            n3022 = local write "Do 0"(w4184) -> ()
          }
          frame 1 {
            n3023 = local write "Do 1"(w4185) -> ()
          }
          frame 2 {
            n3024 = local write "Do 2"(w4186) -> ()
          }
          frame 3 {
            n3025 = local write "Do 3"(w4187) -> ()
          }
          frame 4 {
            n3026 = local write "Do 4"(w4188) -> ()
          }
          frame 5 {
            n3027 = local write "Do 5"(w4189) -> ()
          }
          frame 6 {
            n3028 = local write "Do 6"(w4190) -> ()
          }
          frame 7 {
            n3029 = local write "Do 7"(w4191) -> ()
          }
        }
        n3030 = case shown="1" w4182 {
          tunnel: "PWR" -> [w4192 w4193 w4194 w4195 w4196 w4197 w4198 w4199]
          frame 0, Default {
            n3031 = local write "Do 0"(w4192) -> ()
          }
          frame 1 {
            n3032 = local write "Do 1"(w4193) -> ()
          }
          frame 2 {
            n3033 = local write "Do 2"(w4194) -> ()
          }
          frame 3 {
            n3034 = local write "Do 3"(w4195) -> ()
          }
          frame 4 {
            n3035 = local write "Do 4"(w4196) -> ()
          }
          frame 5 {
            n3036 = local write "Do 5"(w4197) -> ()
          }
          frame 6 {
            n3037 = local write "Do 6"(w4198) -> ()
          }
          frame 7 {
            n3038 = local write "Do 7"(w4199) -> ()
          }
        }
      }
    }
    n3039 = local read "RUN"() -> (w4122:bool)
    n3040 = Or(x=w4122, y="ACQUIRE 3") -> (x .or. y?=w4121:bool)
    n3041 = local read "Set Hz"() -> (w4139:dbl)
    n3042 = Select(t=w4139, s=w4121, f=0.0) -> (s? t:f=w4138:dbl)
    n3043 = local read "st gain"() -> (w4142:string)
    n3044 = local read "DO"() -> (w4143:string)
    n3045 = case shown="True" "Boolean 10" {
      frame False {
      }
      frame True {
        n3046 = local write "Tab Control 8"(enum32{"setup", "calibrate"}."calibrate" ("Tab Control 8")) -> ()
        n3047 = local write "Boolean 10"(FALSE ("Boolean 10")) -> ()
      }
    }
    n3048 = Number To Decimal String(number=w4138) -> (decimal integer string=w4141:string)  [unwired: 1 in]
    n3049 = case shown="True" "Boolean 11" {
      frame False {
      }
      frame True {
        n3050 = local write "Tab Control 8"(enum32{"setup", "calibrate"}."setup" ("Tab Control 8")) -> ()
        n3051 = local write "Boolean 11"(FALSE ("Boolean 11")) -> ()
      }
    }
    n3052 = String Length(string=w4142) -> (length=w4157:i32)
    n3053 = String Length(string=w4143) -> (length=w4145:i32)
    n3054 = String Length(string=w4141) -> (length=w4158:i32)
    n3055 = Subtract(x=4.0, y=w4157) -> (x-y=w4154:dbl)
    n3056 = Subtract(x=3.0, y=w4145) -> (x-y=w4148:dbl)
    n3057 = flat-sequence {
      tunnel: w4168 -> [_]
      frame #0 {
        n3058 = Build Array("Do 0", "Do 1", "Do 2", "Do 3", "Do 4", "Do 5", "Do 6", "Do 7") -> (w4226:bool[])
        n3059 = Boolean Array To Number(Boolean array=w4226) -> (number=w4224:u32)
        n3060 = Add(x=w4224, y=u32 0) -> (x+y=w4222:u32)
        n3061 = Number To Decimal String(number=w4222) -> (decimal integer string=→"DO":string)  [unwired: 1 in]
      }
    }
    n3062 = Subtract(x=3.0, y=w4158) -> (x-y=w4159:dbl)
    n3063 = Replace Substring(3:w4154, 4:w4142, 5:"0000" ("string")) -> (1:w4152:string)  [unwired: 1 in, 1 out]
    n3064 = Replace Substring(3:w4148, 4:w4143, 5:"000" ("string")) -> (1:w4144:string)  [unwired: 1 in, 1 out]
    n3065 = Replace Substring(3:w4159, 4:w4141, 5:"000" ("string")) -> (1:w4153:string)  [unwired: 1 in, 1 out]
    n3066 = Concatenate Strings("*" ("string"), w4153, w4151, w4152, w4151, w4144, "$" ("string")) -> (w4149:string)
    "Stroke_send_Val" <- w4149
    n3067 = local read "RUN"() -> (w4119:bool)
    n3068 = local read "ACQUIRE 3"() -> (w4118:bool)
    n3069 = local read "send"() -> (w4135:bool)
    n3070 = Not Equal?(x=w4137, y=w4149) -> (x != y?=w4150:bool)
    n3071 = Or(x=w4119, y=w4118) -> (x .or. y?=w4117:bool)
    n3072 = And(x=w4135, y=w4117) -> (x .and. y?=w4134:bool)
    n3073 = Or(x=w4150, y=w4134) -> (x .or. y?=w4128:bool)
    n3074 = case shown="False" w4117 {
      frame False {
        "send" <- TRUE ("send")
      }
      frame True {
      }
    }
    n3075 = call "Elapsed Time4"("Time Target (s)"=0.5) -> ("Time has Elapsed"=w4126:bool)  [unwired: 11 in, 7 out]
    n3076 = local read "Din"() -> (w4167:u8[])
    n3077 = Or(x=w4126, y=w4128) -> (x .or. y?=w4127:bool)
    n3078 = local read "Quit"() -> (w4111:bool)
    n3079 = Index Array(array=w4167, index=0) -> (element=w4165:u8)
    n3080 = case shown="True" w4127 {
      tunnel: w4149 -> [_ w4203]
      frame False {
      }
      frame True {
        n3081 = local read "Due Com"() -> (w4204:string[])
        n3082 = Build Array (concatenate)(w4204, w4203) -> (→"Due Com":string[])
        n3083 = local write "send"(FALSE ("send")) -> ()
      }
    }
    n3084 = Number To Boolean Array(number=w4165) -> (Boolean array=w4164:bool[])
    n3085 = Array Size(array=w4164) -> (size(s)=w4163:i32)
    n3086 = Greater Than 0?(x=w4163) -> (x > 0?=w4162:bool)
    n3087 = case shown="True" w4162 {
      tunnel: w4164 -> [_ w4218]
      frame False {
      }
      frame True {
        n3088 = Index Array(array=w4218, index #1=0 ("index"), index #2=1 ("index"), index #3=2 ("index"), index #4=3 ("index"), index #5=4 ("index"), index #6=5 ("index"), index #7=6 ("index"), index #8=7 ("index")) -> (element #1=→"DI 0":bool, element #2=→"DI 1":bool, element #3=→"DI 2":bool, element #4=→"DI 3":bool, element #5=→"DI 4":bool, element #6=→"DI 5":bool, element #7=→"DI 6":bool, element #8=→"DI 7":bool)
      }
    }
  }
  n3089 = Or(x=w29, y=w34) -> (x .or. y?=w41:bool)
  n3090 = control-ref of="new picture"() -> ()  [unwired: 1 out]
  n3091 = Or(x=w48, y=w41) -> (x .or. y?=w38:bool)
  n3092 = Or(x=w38, y=w39) -> (x .or. y?=w30:bool)
  n3093 = while {
    tunnel: [w4273] -> w52
    tunnel: [w4274] -> _
    i -> [w4274]
    stop <- w4273 stop-if-true
    n3094 = local read "PID-out"() -> (w4275:dbl)
    "Horizontal Slider Control" <- w4275
    n3095 = Greater Or Equal?(x=w4275, y=2.0) -> (x >= y?=w4276:bool)
    n3096 = flat-sequence {
      tunnel: w4276 -> [w4284]
      tunnel: w4275 -> [w4287]
      tunnel: [w4285] -> w4282
      tunnel: [w4283] -> w4281
      tunnel: [w4303] -> w4280
      tunnel: w4282 -> [w4303]
      tunnel: w4281 -> [w4300]
      tunnel: [w4300] -> w4279
      tunnel: w4280 -> [w4305]
      tunnel: [w4304] -> w4278
      tunnel: w4279 -> [w4304]
      tunnel: w4278 -> [w4319]
      frame #0 {
        n3097 = case shown="True" w4284 {
          selector: w4284 -> [w4289 _]
          frame False {
            n3098 = local write "HEATER"(w4289) -> ()
          }
          frame True {
            w4291 = TRUE ("data")
            n3099 = local read "CH-HEATER"() -> (w4290:u16)
            n3100 = case shown="2" w4290 {
              tunnel: w4291 -> [w4292 w4293 w4294 w4295 w4296 w4297 w4298 w4299]
              frame 0, Default {
                n3101 = local write "Do 0"(w4292) -> ()
              }
              frame 1 {
                n3102 = local write "Do 1"(w4293) -> ()
              }
              frame 2 {
                n3103 = local write "Do 2"(w4294) -> ()
              }
              frame 3 {
                n3104 = local write "Do 3"(w4295) -> ()
              }
              frame 4 {
                n3105 = local write "Do 4"(w4296) -> ()
              }
              frame 5 {
                n3106 = local write "Do 5"(w4297) -> ()
              }
              frame 6 {
                n3107 = local write "Do 6"(w4298) -> ()
              }
              frame 7 {
                n3108 = local write "Do 7"(w4299) -> ()
              }
            }
            "HEATER" <- w4291
          }
        }
        n3109 = Select(t=w4287, s=w4284, f=0.0) -> (s? t:f=w4283:dbl)
        n3110 = Greater Or Equal?(x=w4287, y=97.0) -> (x >= y?=w4285:bool)
      }
      frame #1 {
        n3111 = Multiply(x=w4300, y=5.0) -> (x*y=w4302:dbl)
        n3112 = Wait (ms)(milliseconds to wait=w4302) -> ()  [unwired: 1 out]
      }
      frame #2 {
        n3113 = case shown="False" w4305 {
          frame False {
            w4306 = FALSE ("data")
            n3114 = local read "CH-HEATER"() -> (w4307:u16)
            n3115 = case shown="4" w4307 {
              tunnel: w4306 -> [w4308 w4309 w4310 w4311 w4312 w4313 w4314 w4315]
              frame 0, Default {
                n3116 = local write "Do 0"(w4308) -> ()
              }
              frame 1 {
                n3117 = local write "Do 1"(w4309) -> ()
              }
              frame 2 {
                n3118 = local write "Do 2"(w4310) -> ()
              }
              frame 3 {
                n3119 = local write "Do 3"(w4311) -> ()
              }
              frame 4 {
                n3120 = local write "Do 4"(w4312) -> ()
              }
              frame 5 {
                n3121 = local write "Do 5"(w4313) -> ()
              }
              frame 6 {
                n3122 = local write "Do 6"(w4314) -> ()
              }
              frame 7 {
                n3123 = local write "Do 7"(w4315) -> ()
              }
            }
            n3124 = local write "HEATER"(w4306) -> ()
          }
          frame True {
          }
        }
      }
      frame #3 {
        n3125 = Subtract(x=100, y=w4319) -> (x-y=w4318:dbl)
        n3126 = Multiply(x=w4318, y=5.0) -> (x*y=w4316:dbl)
        n3127 = Wait (ms)(milliseconds to wait=w4316) -> ()  [unwired: 1 out]
      }
    }
    n3128 = local read "Quit"() -> (w4273:bool)
  }
  n3129 = Or(x=w52, y=w30) -> (x .or. y?=w51:bool)
  n3130 = while {
    tunnel: [w4321] -> w47
    i -> [w4328]
    stop <- w4321 stop-if-true
    n3131 = local read "Quit"() -> (w4321:bool)
    n3132 = Equal To 0?(x=w4328) -> (x = 0?=w4326:bool)
    n3133 = call "Elapsed Time3"("Time Target (s)"=45.0, "Auto Reset"=TRUE) -> ("Time has Elapsed"=w4325:bool)  [unwired: 10 in, 7 out]
    n3134 = Wait (ms)(milliseconds to wait=u32 50) -> ()  [unwired: 1 out]
    n3135 = Or(x=w4325, y=w4326) -> (x .or. y?=w4327:bool)
    n3136 = case shown="True" w4327 {
      frame False {
      }
      frame True {
        n3137 = call <vilib>:"System Exec.vi"("run minimized? (F)"=TRUE, "error in (no error)"="error in (no error)", "command line"="powercfg.exe -change -monitor-timeout-ac 0") -> ("error out"=w4339:errorcluster)  [unwired: 5 in, 3 out]
        n3138 = call <vilib>:"System Exec.vi"("run minimized? (F)"=TRUE, "error in (no error)"=w4339, "command line"="powercfg.exe -change -disk-timeout-ac 0") -> ("error out"=w4338:errorcluster)  [unwired: 5 in, 3 out]
        n3139 = call <vilib>:"System Exec.vi"("run minimized? (F)"=TRUE, "error in (no error)"=w4338, "command line"="powercfg.exe -change -standby-timeout-ac 0") -> ("error out"=w4337:errorcluster)  [unwired: 5 in, 3 out]
        n3140 = call <vilib>:"System Exec.vi"("run minimized? (F)"=TRUE, "error in (no error)"=w4337, "command line"="powercfg.exe -change -hibernate-timeout-ac 0") -> ("error out"=w4336:errorcluster)  [unwired: 5 in, 3 out]
        n3141 = call <vilib>:"Simple Error Handler.vi"("error in (no error)"=w4336) -> ("error out"=w4342:errorcluster)  [unwired: 4 in, 4 out]
        n3142 = call <vilib>:"Clear Errors.vi"("error in (no error)"=w4342) -> ("error out"=→"error out":errorcluster)  [unwired: 5 in, 1 out]
      }
    }
  }
  n3143 = Compound Arithmetic op=OR(w50, w51, w47) -> (w49:bool)
  n3144 = flat-sequence {
    tunnel: w49 -> [_]
    tunnel: [w4344] -> w5
    tunnel: w5 -> [_]
    frame #0 {
      n3145 = call "CLOSE CONNECTION.vi"() -> ("error out"=w4344:errorcluster)  [unwired: 11 in]
    }
    frame #1 {
      n3146 = Quit LabVIEW(quit? (T)=TRUE) -> ()
      n3147 = local write "Quit"(FALSE ("EXIT")) -> ()
    }
  }
  n3148 = property on="Heater Button" class="Bool (strict)"("Visible"=TRUE) -> ()  [unwired: 2 in, 2 out]
  n3149 = disable-structure shown="Disabled" {
    disable-tunnel: _ -> [w4350 _]
    disable-tunnel: _ -> [w4347 _]
    disable-tunnel: _ -> [w4348 _]
    frame Disabled {
      n3150 = disable-structure shown="Disabled" {
        disable-tunnel: [w4357 _] -> w4349
        frame Disabled {
          n3151 = while {
            shift-right: [w4399] -> w4355
            shift-left: errorcluster {"status"=TRUE, "code"=0, "source"="Init"} ("error out") -> [w4364]
            shift-right: [w4398] -> w4354
            shift-left: _ -> [w4365]
            shift-right: [w4397] -> _
            shift-left: "" -> [w4396]
            tunnel: [w4358] -> w4357
            shift-right: ["Set Rh"] -> _
            shift-left: 0.0 ("Set Rh") -> [w4390]
            tunnel: [w4367] -> _
            i -> [w4367]
            stop <- w4358 stop-if-true
            n3152 = flat-sequence {
              tunnel: w4364 -> [w4402]
              tunnel: [w4402] -> w4363
              frame #0 {
                n3153 = Wait (ms)(milliseconds to wait=u32 200) -> ()  [unwired: 1 out]
              }
            }
            n3154 = local read "Com Port 3"() -> (w4366:refnum<visa-resource-name>)
            n3155 = local read "Humidity Str Rec"() -> (w4368:string)
            n3156 = Not Equal?(x="Set Rh", y=w4390) -> (x != y?=w4395:bool)
            n3157 = Number To Decimal String(number="Set Rh") -> (decimal integer string=w4393:string)  [unwired: 1 in]
            n3158 = Not Equal?(x=w4366, y=w4365) -> (x != y?=w4361:bool)
            n3159 = Concatenate Strings("#setPoint00" ("string"), w4393) -> (w4394:string)
            n3160 = case shown="False" w4395 {
              tunnel: w4394 -> [_ w4414]
              frame False {
                n3161 = local read "Humidity"() -> (w4411:bool)
                n3162 = case shown="True" w4411 {
                  frame False {
                    n3163 = local write "Humidity Str Send"("stop" ("Humidity Str Send")) -> ()
                  }
                  frame True {
                    n3164 = local write "Humidity Str Send"("start" ("Humidity Str Send")) -> ()
                  }
                }
              }
              frame True {
                n3165 = local write "Humidity Str Send"(w4414) -> ()
              }
            }
            n3166 = Or(x=w4361, y="Re-Initialise") -> (x .or. y?=w4360:bool)
            n3167 = String Subset(string=w4368, offset (0)=7) -> (substring=w4383:string)  [unwired: 1 in]
            n3168 = Match Pattern(string=w4368, regular expression="?") -> (offset past match=w4386:i32)  [unwired: 1 in, 3 out]
            n3169 = Match Pattern(string=w4368, regular expression="v") -> (offset past match=w4389:i32)  [unwired: 1 in, 3 out]
            n3170 = case shown="True" w4360 {
              tunnel: w4363 -> [w4400 _]
              tunnel: [w4400 errorcluster {"status"=TRUE, "code"=0, "source"="Init"} ("error out")] -> w4362
              frame False {
              }
              frame True {
              }
            }
            n3171 = Equal?(x=w4386, y=-1) -> (x = y?=w4370:bool)
            n3172 = Match Pattern(string=w4383, regular expression="g") -> (after substring=w4384:string, offset past match=w4375:i32)  [unwired: 1 in, 2 out]
            n3173 = Match Pattern(string=w4383, regular expression="y") -> (after substring=w4382:string, offset past match=w4376:i32)  [unwired: 1 in, 2 out]
            n3174 = Greater?(x=w4376, y=w4375) -> (0:w4381:bool)
            n3175 = Greater Or Equal To 0?(x=w4376) -> (x >= 0?=w4373:bool)
            n3176 = Greater Or Equal To 0?(x=w4375) -> (x >= 0?=w4374:bool)
            n3177 = Or(x=w4373, y=w4374) -> (x .or. y?=w4372:bool)
            n3178 = Greater Or Equal To 0?(x=w4389) -> (x >= 0?=w4371:bool)
            n3179 = Select(t=w4382, s=w4381, f=w4384) -> (s? t:f=w4377:string)
            n3180 = case shown="Error" w4362 {
              selector: w4362 -> [w4427 w4473]
              tunnel: [w4425 w4466] -> w4399
              tunnel: w4365 -> [w4428 w4472]
              tunnel: [w4426 w4475] -> w4398
              tunnel: w4396 -> [w4415 w4474]
              tunnel: [w4422 w4474] -> w4397
              frame No Error {
                n3181 = call "Elapsed Time7"() -> ("Time has Elapsed"=w4421:bool)  [unwired: 12 in, 7 out]
                n3182 = Not Equal?(x="Humidity Str Send", y=w4415) -> (x != y?=w4417:bool)
                n3183 = Or(x=w4417, y=w4421) -> (x .or. y?=w4420:bool)
                n3184 = Select(t="Humidity Str Send", s=w4417, f="vals" ("regular expression")) -> (s? t:f=w4416:string)
                n3185 = Or(x=w4420, y="Send") -> (x .or. y?=w4424:bool)
                n3186 = case shown="True" w4424 {
                  tunnel: [w4431 w4436] -> w4425
                  tunnel: w4428 -> [w4430 w4444]
                  tunnel: w4427 -> [w4431 w4443]
                  tunnel: [w4430 w4437] -> w4426
                  tunnel: w4416 -> [_ w4442]
                  tunnel: [w4429 w4433] -> w4422
                  tunnel: "Humidity Str Send" -> [_ w4434]
                  tunnel: w4417 -> [_ w4435]
                  tunnel: w4415 -> [w4429 w4432]
                  frame False {
                  }
                  frame True {
                    n3187 = flat-sequence {
                      tunnel: w4444 -> [w4452]
                      tunnel: w4443 -> [w4451]
                      tunnel: w4442 -> [w4448]
                      tunnel: [w4450] -> w4441
                      tunnel: [w4449] -> w4440
                      tunnel: w4441 -> [w4455]
                      tunnel: w4440 -> [w4454]
                      tunnel: [w4455] -> w4439
                      tunnel: [w4454] -> w4438
                      tunnel: w4439 -> [w4462]
                      tunnel: w4438 -> [w4461]
                      tunnel: [w4460] -> w4437
                      tunnel: [w4459] -> w4436
                      frame #0 {
                        n3188 = local write "Ser Led"(TRUE ("Boolean 4")) -> ()
                        n3189 = Concatenate Strings(w4448, "\r") -> (w4447:string)
                        n3190 = VISA Write(VISA resource name=w4452, write buffer=w4447, error in (no error)=w4451) -> (VISA resource name out=w4450:refnum<visa-resource-name>, error out=w4449:errorcluster)  [unwired: 1 out]
                      }
                      frame #1 {
                        n3191 = Wait (ms)(milliseconds to wait="wait") -> ()  [unwired: 1 out]
                      }
                      frame #2 {
                        w4457 = FALSE ("Send")
                        n3192 = property class="Instr"(reference=w4462, error in=w4461) -> (reference out=w4463:refnum<visa-resource-name>, error out=w4464:errorcluster, "Serial Settings:Number of Bytes at Serial Port"=w4456:u32)
